vi "Intensity Graph Vertical Linecut.vi"(8 "error in (no error)":errorcluster, 9 "width (vertical)":dbl, 10 "Intensity Data":dbl[][](array[numeric]), 11 "graph_utilities in":refnum<class "graph_utilities.lvclass">) -> (0 "error out":errorcluster, 2 "XY-data vertical":cluster{"Intensity Data":dbl[], "Array":dbl[]}, 3 "graph_utilities out":refnum<class "graph_utilities.lvclass">)   [LabVIEW 2016, in "graph_utilities.lvclass"]
uses:
  graph_utilities.lvclass
  graph_utilities.lvclass/graph_utilities.ctl
  <vilib>/Analysis/baseanly.llb/A x Vector.vi
  <vilib>/Analysis/NI_AALBase.lvlib
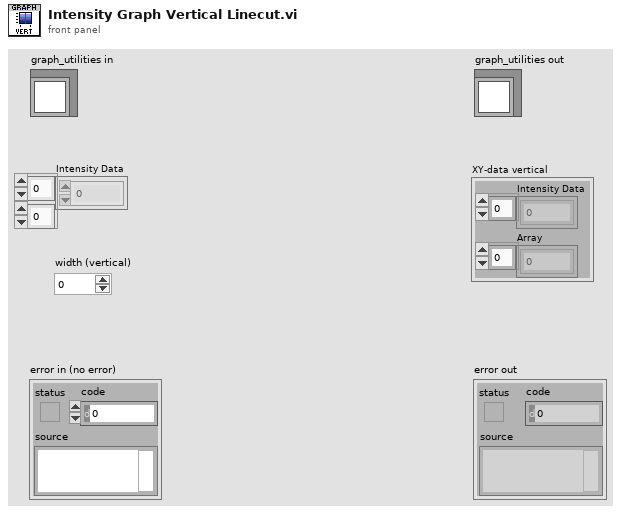
[diagram p1: front panel]
types:
  T1 = typedef "LVPointDoubleTypeDef.ctl" = cluster{"Cursor X":dbl, "Cursor Y":dbl}
  T2 = typedef "LVOffsetAndMultiplierTypeDef.ctl" = cluster{"Offset":dbl, "Multiplier":dbl}
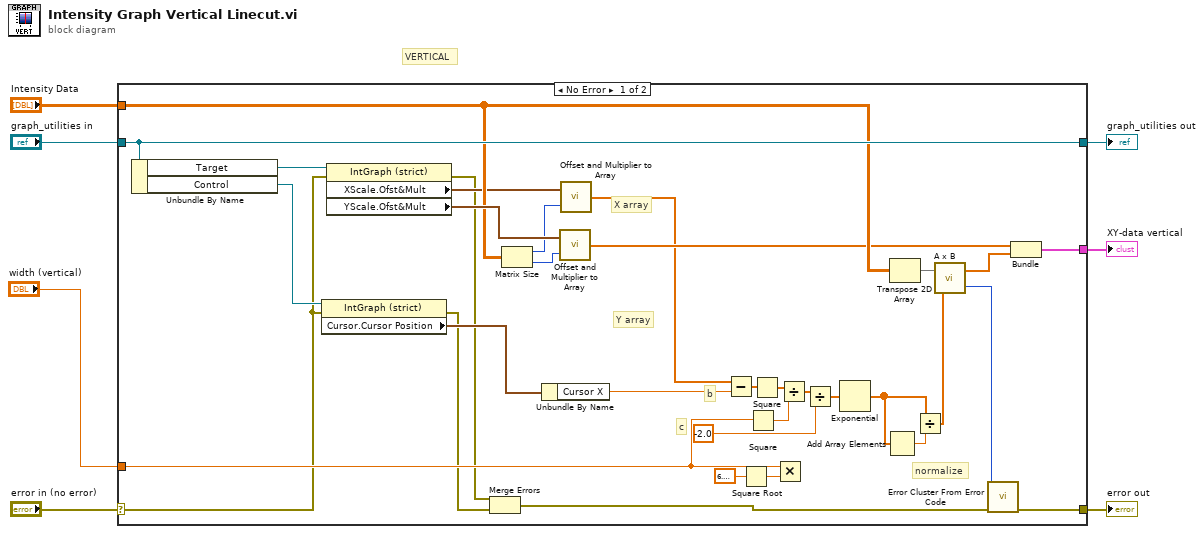
[diagram p0: block diagram]
diagram:
  # "VERTICAL"
  n1 = case shown="No Error" "error in (no error)" {
    selector: "error in (no error)" -> [w12 w42]
    tunnel: [w15 w42] -> w6
    tunnel: [w40 w41] -> w4
    tunnel: "graph_utilities in" -> [w40 w41]
    tunnel: "Intensity Data" -> [w34 _]
    tunnel: [w22 _] -> w1
    tunnel: "width (vertical)" -> [w18 _]
    frame No Error {
      # "normalize"
      # "b"
      # "c"
      # "X array"
      # "Y array"
      n2 = Unbundle By Name(w40) -> ("Target"=w20:refnum<vi>, "Control"=w13:refnum<vi>)
      n3 = property on="Property Node" class="IntGraph (strict)"(reference=w13, error in=w12) -> (error out=w8:errorcluster, "Cursor.Cursor Position"=w11:T1)  [unwired: 1 out]
      n4 = property on="Property Node" class="IntGraph (strict)"(reference=w20, error in=w12) -> (error out=w9:errorcluster, "XScale.Ofst&Mult"=w16:T2, "YScale.Ofst&Mult"=w39:T2)  [unwired: 1 out]
      n5 = Merge Errors(w9, w8) -> (w10:errorcluster)
      n6 = Matrix Size(0:w34) -> (1:w35:i32, 2:w38:i32)
      n7 = Unbundle By Name(w11) -> ("Cursor X"=w36:dbl)
      n8 = call "Offset and Multiplier to Array.vi"("Size"=w38, "Offset and Multiplier"=w39) -> ("Array"=w21:dbl[])
      n9 = call "Offset and Multiplier to Array.vi"("Size"=w35, "Offset and Multiplier"=w16) -> ("Array"=w19:dbl[])
      n10 = Subtract(x=w19, y=w36) -> (x-y=w31:dbl[])
      n11 = Square Root(x=6.283185307179586) -> (sqrt(x)=w28:dbl)
      n12 = Square(x=w18) -> (x^2=w27:dbl)
      n13 = Square(x=w31) -> (x^2=w30:dbl[])
      n14 = Multiply(x=w18, y=w28) -> ()  [unwired: 1 out]
      n15 = Divide(x=w30, y=w27) -> (x/y=w26:dbl[])
      n16 = Divide(x=w26, y=-2.0 ("value")) -> (x/y=w24:dbl[])
      n17 = Exponential(1:w24) -> (0:w17:dbl[])
      n18 = Add Array Elements(numeric array=w17) -> (sum=w23:dbl)
      n19 = Transpose 2D Array(2D array=w34) -> (transposed array=w37:dbl[][])
      n20 = Divide(x=w17, y=w23) -> (x/y=w32:dbl[])
      n21 = call-poly <vilib>:"A x B.vi"("Vector"=w32, "A"=w37) -> ("error"=w14:i32, "A x Vector"=w33:dbl[])
      n22 = call <vilib>:"Error Cluster From Error Code.vi"("error in (no error)"=w10, "error code (0)"=w14) -> ("error out"=w15:errorcluster)  [unwired: 7 in]
      n23 = Bundle("Array"=w21, "A x Vector"=w33) -> (w22:cluster{"Array":dbl[], "A x Vector":dbl[]})  [unwired: 1 in]
    }
    frame Error {
    }
  }
  "error out" <- w6
  "graph_utilities out" <- w4
  "XY-data vertical" <- w1
